vi "SMU simple tester.vi"() -> ()   [LabVIEW 2021]
uses:
  ctls/SMU status.ctl
  Source meter.lvlib
  <instrlib>/Keithley 2450/Keithley 2450.lvlib
  <userlib>/_MGI/1D Array/MGI Average/MGI Average (DBL[]).vi
  ctls/SMU settings.ctl
panel:
  out "Waveform Chart 2":dbl(graph)
  in  "Refresh Button":bool
  in  "VISA resource name 2":refnum<visa-resource-name>
  out "error":errorcluster
  out "Event Logger":string[](array[string])
  out "data":dbl[](array[numeric])
  out "SMU status":T1 {"Measure Function" items=["Volts", "Current", "Auto Resistance", "Manual Resistance", "Digitize Voltage", "Digitize Current"]; "Source Mode" items=["Voltage", "Current"]}
  out "Waveform Chart":dbl(graph)
  in  "Measurement settings":T2={"Source Mode "=1, "Source Level"=0.001, "Source Limit"=0.1, "Measure Function"=0, "Remote sense"=FALSE, "Clear buffer?"=FALSE, "Beep"=FALSE, "High Capacity"=FALSE, "Terminals"=0, "PLCs"=1.0, "Fast measurement"=FALSE} {"Measure Function" items=["Volts", "Current", "Auto Resistance", "Manual Resistance", "Digitize Voltage", "Digitize Current"]; "Source Mode" items=["Voltage", "Current"]; "Terminals" items=["Front", "Rear"]}
  in  "Disconnect":bool
  in  "Setup measuerment":bool
  in  "Start measurment":bool
  in  "Stop measurement":bool
  in  "End":bool
  in  "Connect":bool
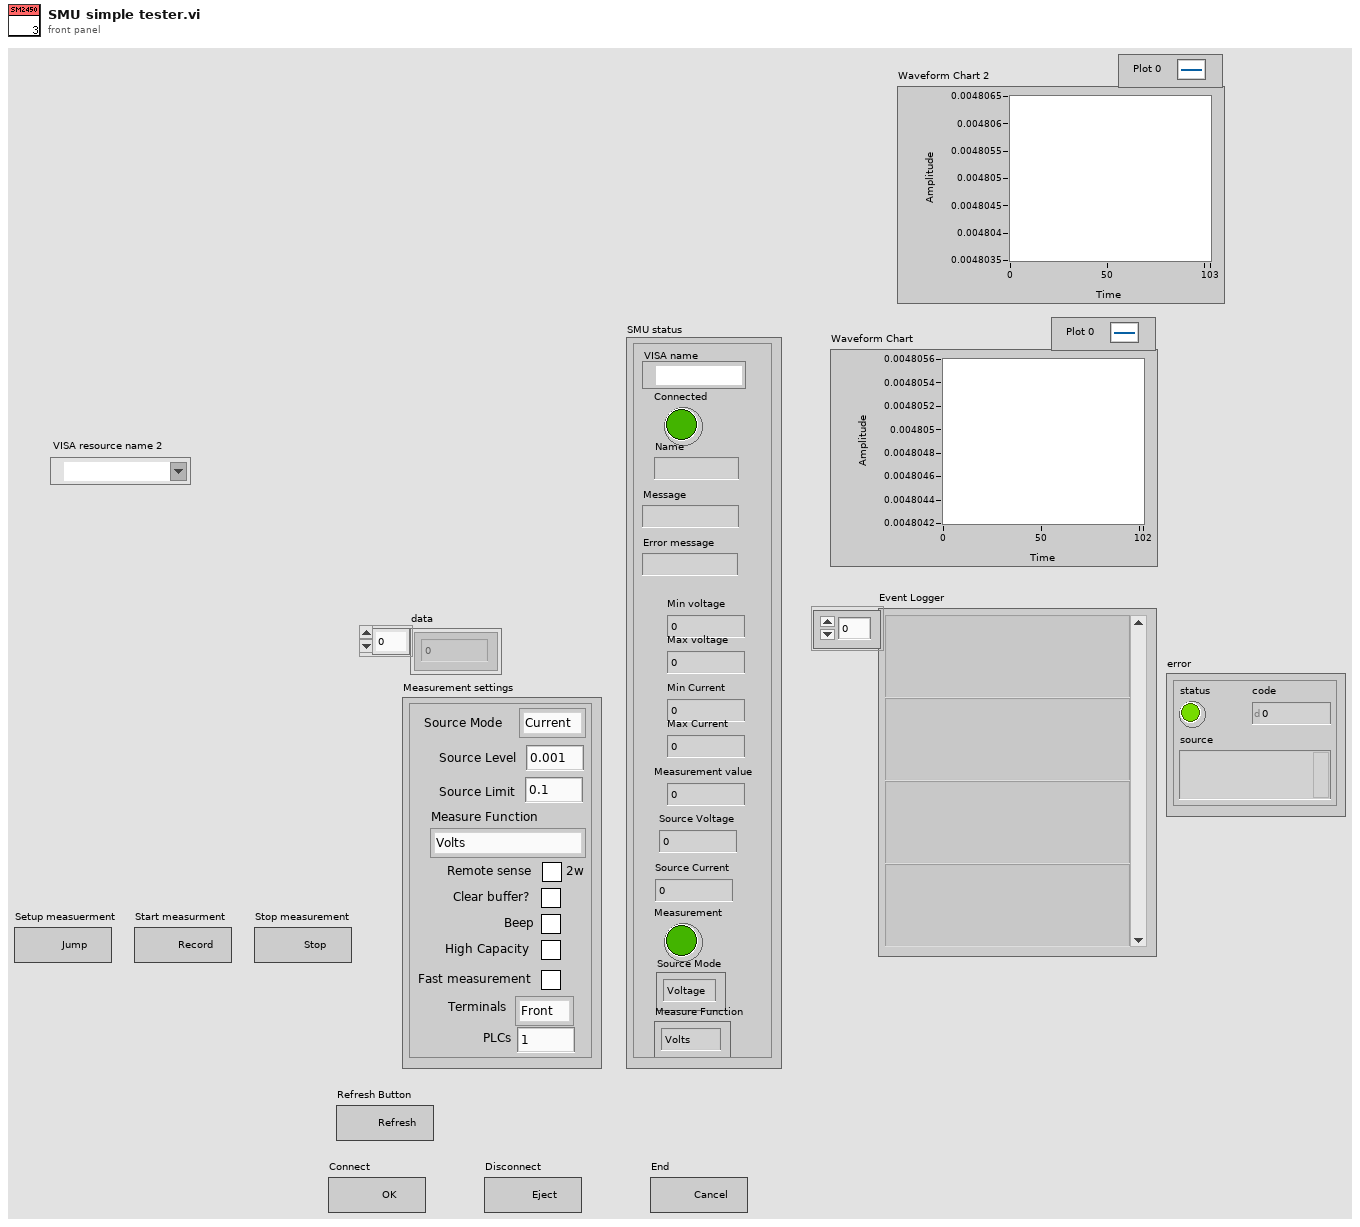
[diagram p1: front panel]
types:
  T1 = typedef "Source meter.lvlib/SMU status.ctl" = cluster{"VISA name":refnum<visa-resource-name>, "Connected":bool, "Name":string, "Message":string, "Error message":string, "Min voltage":dbl, "Max voltage":dbl, "Min Current":dbl, "Max Current":dbl, "Measurement value":dbl, "Source Voltage":dbl, "Measurement":bool, "Source Current":dbl, "Source Mode":u16, "Measure Function":u16}
  T2 = typedef "SMU settings.ctl" = cluster{"Source Mode ":u16, "Source Level":dbl, "Source Limit":dbl, "Measure Function":u16, "Remote sense":bool, "Clear buffer?":bool, "Beep":bool, "High Capacity":bool, "Terminals":u16, "PLCs":dbl, "Fast measurement":bool}
  T3 = cluster{"status":bool, "code":bool, "source":bool}
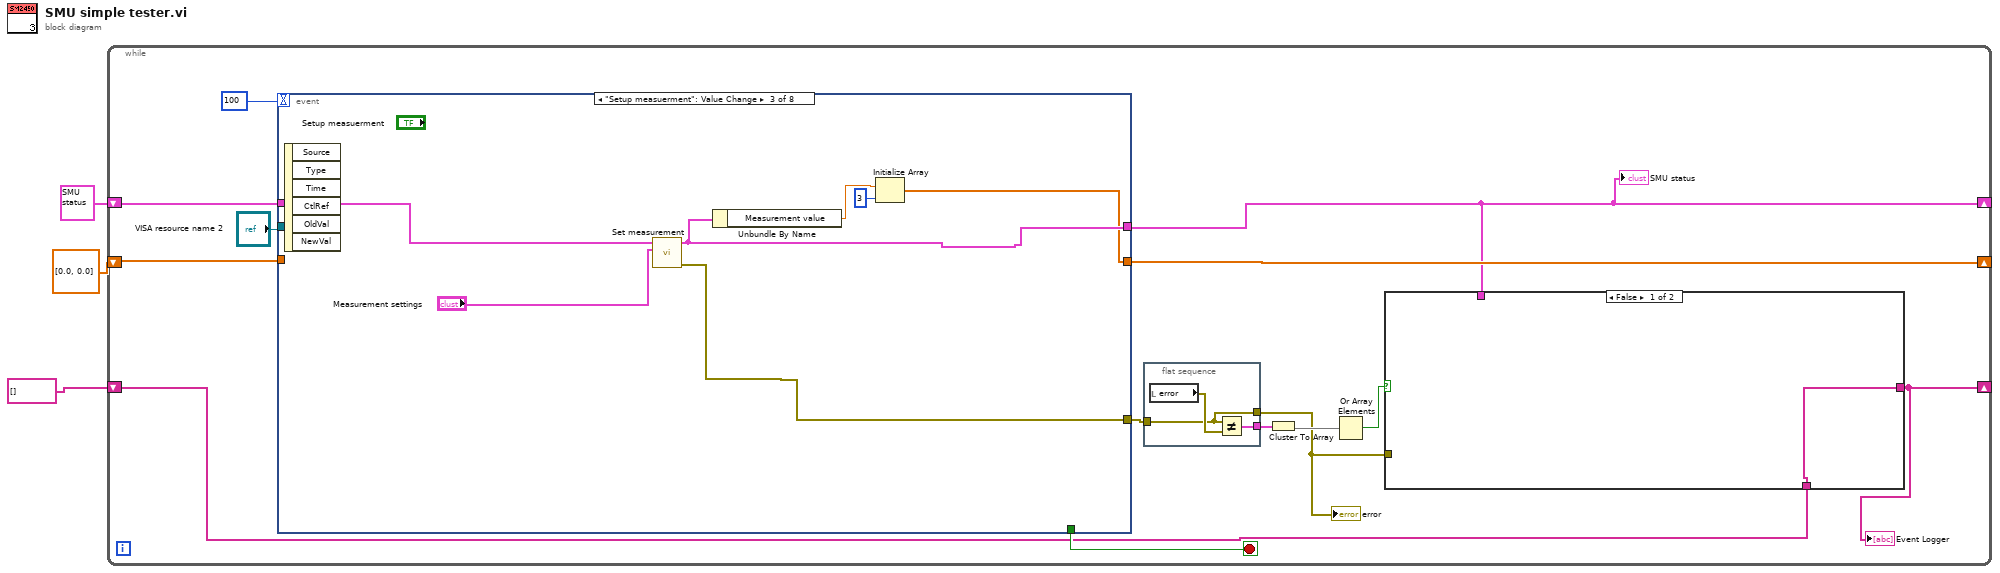
[diagram p0: block diagram]
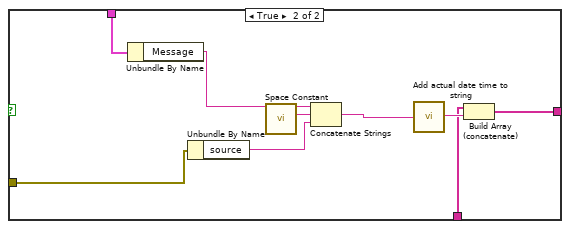
[diagram p2: hidden frame]
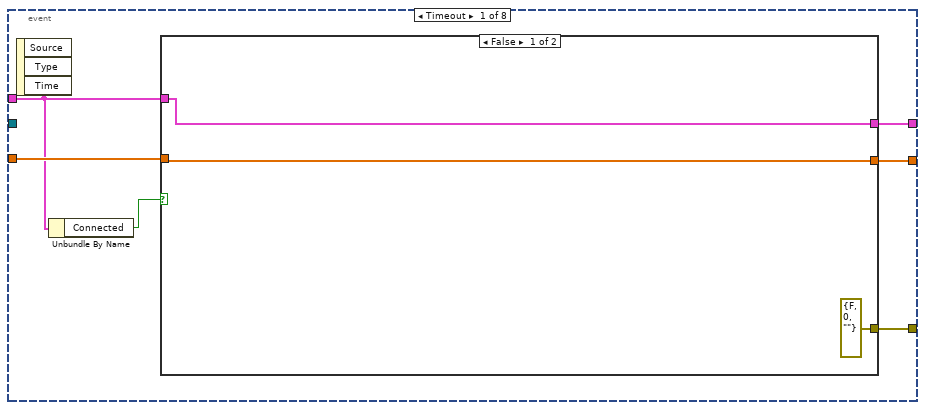
[diagram p3: hidden frame]
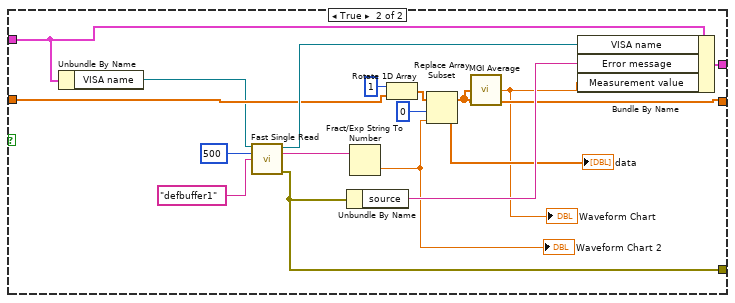
[diagram p4: hidden frame]
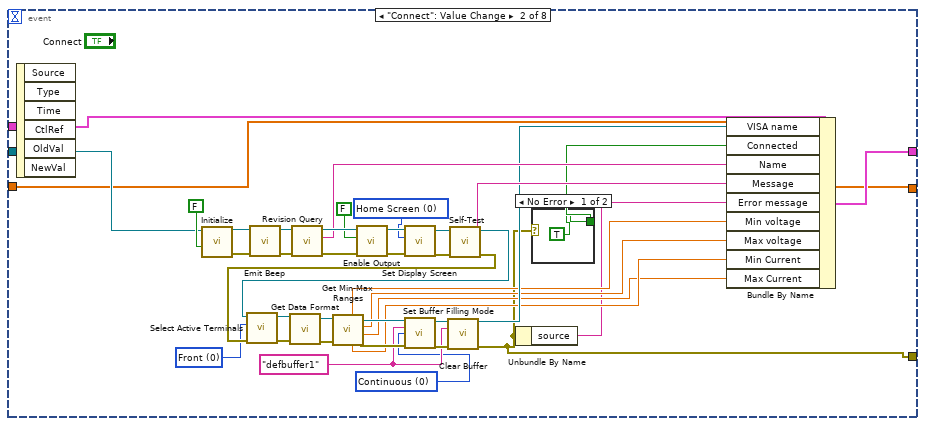
[diagram p5: hidden frame]
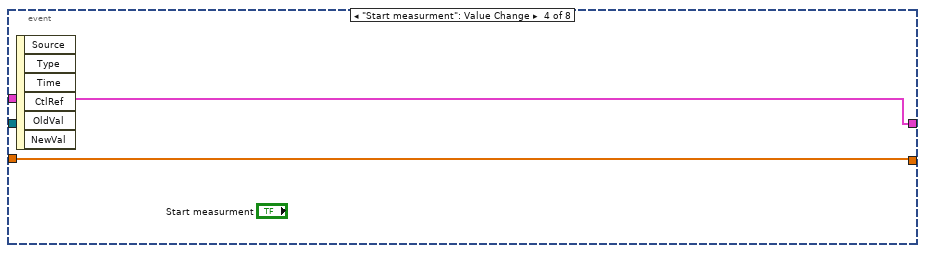
[diagram p7: hidden frame]
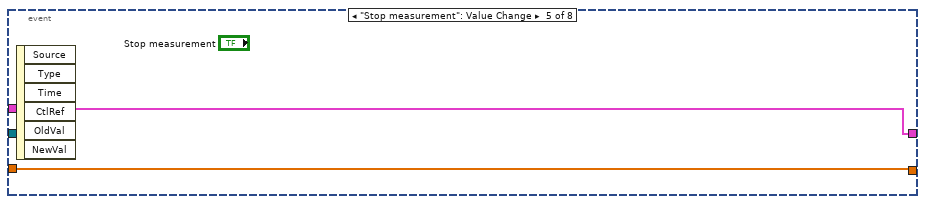
[diagram p8: hidden frame]
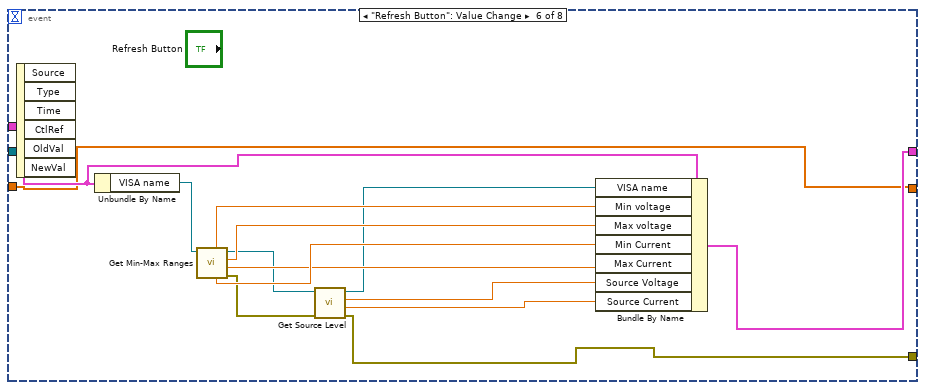
[diagram p9: hidden frame]
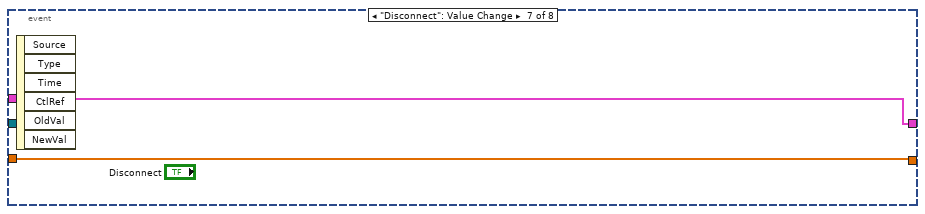
[diagram p10: hidden frame]
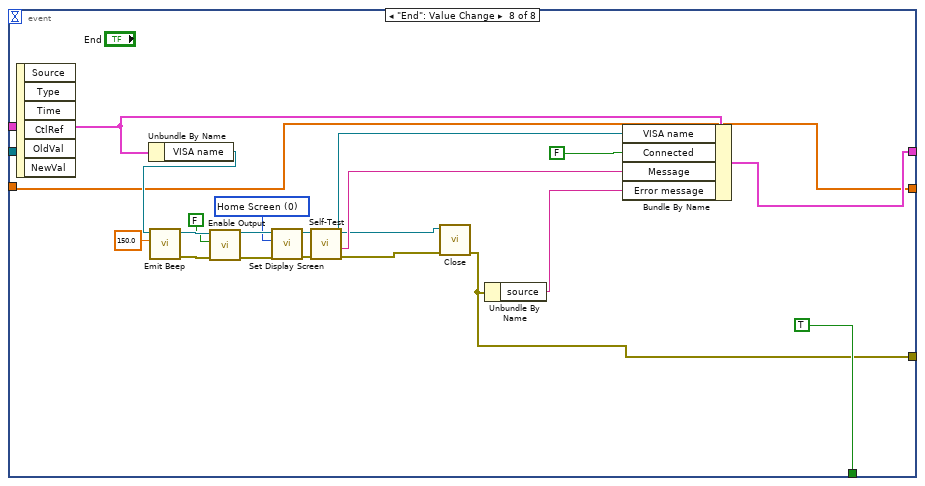
[diagram p11: hidden frame]
diagram:
  n1 = while {
    shift-right: [w4] -> _
    shift-left: T1 {"VISA name"="", "Connected"=FALSE, "Name"="", "Message"="", "Error message"="", "Min voltage"=0.0, "Max voltage"=0.0, "Min Current"=0.0, "Max Current"=0.0, "Measurement value"=0.0, "Source Voltage"=0.0, "Measurement"=FALSE, "Source Current"=0.0, "Source Mode"=0, "Measure Function"=0} ("SMU status") -> [w15]
    shift-right: [w13] -> _
    shift-left: dbl[] [0.0, 0.0] -> [w14]
    shift-right: [w6] -> _
    shift-left: string[] [] ("Event Logger") -> [w5]
    stop <- w16 stop-if-true
    n2 = event shown="[2] \"Setup measuerment\": Value Change" {
      selector: _ -> [_ _ _ _ _ _ _ _]
      dyn-events: _ -> [_ _ _ _ _ _ _ _]
      timeout: 100 -> [_ _ _ _ _ _ _ _]
      tunnel: [_ _ _ _ _ _ _ TRUE] -> w16
      tunnel: "VISA resource name 2" -> [_ w58 _ _ _ _ _ _]
      tunnel: w15 -> [w33 w59 w101 w105 w107 w111 w122 w127]
      tunnel: [w36 w60 w99 w105 w107 w110 w122 w126] -> w4
      tunnel: w14 -> [w35 w57 _ w104 w106 w109 w123 w125]
      tunnel: [w34 w57 w98 w104 w106 w109 w123 w125] -> w13
      tunnel: [w31 w56 w97 _ _ w108 _ w124] -> w11
      event Timeout {
        n3 = event-data() -> ()  [unwired: 1 in, 3 out]
        n4 = Unbundle By Name(w33) -> ("Connected"=w32:bool)
        n5 = case shown="False" w32 {
          tunnel: [w39 w47] -> w36
          tunnel: w35 -> [w38 w46]
          tunnel: [w38 w42] -> w34
          tunnel: w33 -> [w39 w45]
          tunnel: [errorcluster {"status"=FALSE, "code"=0, "source"=""} ("error out") w43] -> w31
          frame False {
          }
          frame True {
            n6 = Unbundle By Name(w45) -> ("VISA name"=w44:refnum<visa-resource-name>)
            n7 = call "Fast Single Read.vi"("VISA resource name"=w44, "Timeout (10000 ms)"=500, "Buffer Name (defbuffer1)"="defbuffer1") -> ("VISA resource name out"=w55:refnum<visa-resource-name>, "Data out"=w54:string, "error out"=w43:errorcluster)  [unwired: 10 in]
            n8 = Unbundle By Name(w43) -> ("source"=w53:string)
            n9 = Fract/Exp String To Number(string=w54) -> (number=w40:dbl)  [unwired: 3 in, 1 out]
            "Waveform Chart 2" <- w40
            n10 = Rotate 1D Array(1:w46, 2:1 ("n")) -> (0:w52:dbl[])
            n11 = Replace Array Subset(array=w52, new element=w40, index=0) -> (w42:dbl[])
            "data" <- w42
            n12 = call-poly <userlib>:"MGI Average.vi"("Double[]"=w42) -> ("Average"=w41:dbl)  [unwired: 1 in]
            "Waveform Chart" <- w41
            n13 = Bundle By Name(cluster=w45, "VISA name"=w55, "Error message"=w53, "Measurement value"=w41) -> (w47:T1)
          }
        }
      }
      event "Connect": Value Change {
        w66 = "defbuffer1" ("Buffer Name (defbuffer1)")
        w63 = u16 0 items=["Front", "Rear"] ("Active Terminals (0: Front)")
        w64 = u16 0 items=["Home Screen", "Source Screen", "Plot Screen", "User-defined Screen", "Statistics Screen", "Settings Screen", "Graph Screen", "Data sheet Screen"] ("Screen Home")
        w65 = u16 0 items=["Continuous", "Once"] ("Fill Type")
        n14 = event-data() -> ()  [unwired: 1 in, 6 out]
        n15 = call <instrlib>:"Initialize.vi"("Reset (True)"=FALSE, "VISA resource name"=w58) -> ("error out"=w94:errorcluster, "VISA resource name out"=w95:refnum<visa-resource-name>)  [unwired: 8 in]
        n16 = call <instrlib>:"Emit Beep.vi"("error in (no error)"=w94, "VISA resource name"=w95) -> ("error out"=w92:errorcluster, "VISA resource name out"=w93:refnum<visa-resource-name>)  [unwired: 8 in]
        n17 = call <instrlib>:"Revision Query.vi"("error in (no error)"=w92, "VISA resource name"=w93) -> ("error out"=w90:errorcluster, "Instrument Driver Revision"=w89:string, "VISA resource name out"=w91:refnum<visa-resource-name>)  [unwired: 6 in, 1 out]
        n18 = call <instrlib>:"Enable Output.vi"("error in (no error)"=w90, "Enable Output (T: Enable)"=FALSE, "VISA resource name"=w91) -> ("error out"=w87:errorcluster, "VISA resource name out"=w88:refnum<visa-resource-name>)  [unwired: 7 in]
        n19 = call <instrlib>:"Set Display Screen.vi"("error in (no error)"=w87, "Screen Home"=w64, "VISA resource name"=w88) -> ("error out"=w84:errorcluster, "VISA resource name out"=w85:refnum<visa-resource-name>)  [unwired: 7 in]
        n20 = call <instrlib>:"Self-Test.vi"("error in (no error)"=w84, "VISA resource name"=w85) -> ("error out"=w68:errorcluster, "Self-Test Result Message"=w86:string, "VISA resource name out"=w69:refnum<visa-resource-name>)  [unwired: 6 in, 1 out]
        n21 = call <instrlib>:"Select Active Terminals.vi"("error in (no error)"=w68, "Active Terminals (0: Front)"=w63, "VISA resource name"=w69) -> ("error out"=w82:errorcluster, "VISA resource name out"=w83:refnum<visa-resource-name>)  [unwired: 7 in]
        n22 = call <instrlib>:"Get Data Format.vi"("VISA resource name"=w83, "error in (no error)"=w82) -> ("VISA resource name out"=w81:refnum<visa-resource-name>, "error out"=w80:errorcluster)  [unwired: 11 in, 1 out]
        n23 = call <instrlib>:"Get Min-Max Ranges.vi"("error in (no error)"=w80, "VISA resource name"=w81) -> ("error out"=w78:errorcluster, "I Max"=w71:dbl, "V Max"=w73:dbl, "VISA resource name out"=w79:refnum<visa-resource-name>, "I Min"=w72:dbl, "V Min"=w74:dbl)  [unwired: 4 in]
        n24 = call <instrlib>:"Set Buffer Filling Mode.vi"("VISA resource name"=w79, "Buffer Name (defbuffer1)"=w66, "Fill Type"=w65, "error in (no error)"=w78) -> ("VISA resource name out"=w77:refnum<visa-resource-name>, "error out"=w76:errorcluster)  [unwired: 10 in]
        n25 = call <instrlib>:"Clear Buffer.vi"("VISA resource name"=w77, "Buffer Name (defbuffer1)"=w66, "error in (no error)"=w76) -> ("VISA resource name out"=w75:refnum<visa-resource-name>, "error out"=w56:errorcluster)  [unwired: 11 in]
        n26 = Unbundle By Name(w56) -> ("source"=w70:string)
        n27 = case shown="No Error" w56 {
          tunnel: [TRUE ("Connected") _] -> w67
          frame No Error {
          }
          frame Error {
          }
        }
        n28 = Bundle By Name(cluster=w59, "VISA name"=w75, "Connected"=w67, "Name"=w89, "Message"=w86, "Error message"=w70, "Min voltage"=w74, "Max voltage"=w73, "Min Current"=w72, "Max Current"=w71) -> (w60:T1)
      }
      event "Setup measuerment": Value Change {
        n29 = event-data() -> ()  [unwired: 1 in, 6 out]
        n30 = call "Set measurement.vi"("Measurement settings"="Measurement settings", "SMU status in"=w101) -> ("error out"=w97:errorcluster, "SMU status out"=w99:T1)  [unwired: 8 in]
        n31 = Unbundle By Name(w99) -> ("Measurement value"=w103:dbl)
        n32 = Initialize Array(w103, 3 ("dimension size")) -> (w98:dbl[])
      }
      event "Start measurment": Value Change {
        n33 = event-data() -> ()  [unwired: 1 in, 6 out]
      }
      event "Stop measurement": Value Change {
        n34 = event-data() -> ()  [unwired: 1 in, 6 out]
      }
      event "Refresh Button": Value Change {
        n35 = event-data() -> ()  [unwired: 1 in, 6 out]
        n36 = Unbundle By Name(w111) -> ("VISA name"=w121:refnum<visa-resource-name>)
        n37 = call <instrlib>:"Get Min-Max Ranges.vi"("VISA resource name"=w121) -> ("error out"=w114:errorcluster, "I Max"=w117:dbl, "V Max"=w119:dbl, "VISA resource name out"=w116:refnum<visa-resource-name>, "I Min"=w118:dbl, "V Min"=w120:dbl)  [unwired: 5 in]
        n38 = call <instrlib>:"Get Source Level.vi"("error in (no error)"=w114, "VISA resource name"=w116) -> ("error out"=w108:errorcluster, "Current Level Out"=w113:dbl, "Voltage Level Out"=w112:dbl, "VISA resource name out"=w115:refnum<visa-resource-name>)  [unwired: 6 in]
        n39 = Bundle By Name(cluster=w111, "VISA name"=w115, "Min voltage"=w120, "Max voltage"=w119, "Min Current"=w118, "Max Current"=w117, "Source Voltage"=w112, "Source Current"=w113) -> (w110:T1)
      }
      event "Disconnect": Value Change {
        n40 = event-data() -> ()  [unwired: 1 in, 6 out]
      }
      event "End": Value Change {
        w130 = u16 0 items=["Home Screen", "Source Screen", "Plot Screen", "User-defined Screen", "Statistics Screen", "Settings Screen", "Graph Screen", "Data sheet Screen"] ("Screen Home")
        n41 = event-data() -> ()  [unwired: 1 in, 6 out]
        n42 = Unbundle By Name(w127) -> ("VISA name"=w133:refnum<visa-resource-name>)
        n43 = call <instrlib>:"Emit Beep.vi"("Beep Frequency (300)"=150.0, "VISA resource name"=w133) -> ("error out"=w141:errorcluster, "VISA resource name out"=w142:refnum<visa-resource-name>)  [unwired: 8 in]
        n44 = call <instrlib>:"Enable Output.vi"("error in (no error)"=w141, "Enable Output (T: Enable)"=FALSE, "VISA resource name"=w142) -> ("error out"=w139:errorcluster, "VISA resource name out"=w140:refnum<visa-resource-name>)  [unwired: 7 in]
        n45 = call <instrlib>:"Set Display Screen.vi"("error in (no error)"=w139, "Screen Home"=w130, "VISA resource name"=w140) -> ("error out"=w136:errorcluster, "VISA resource name out"=w137:refnum<visa-resource-name>)  [unwired: 7 in]
        n46 = call <instrlib>:"Self-Test.vi"("error in (no error)"=w136, "VISA resource name"=w137) -> ("error out"=w134:errorcluster, "Self-Test Result Message"=w138:string, "VISA resource name out"=w135:refnum<visa-resource-name>)  [unwired: 6 in, 1 out]
        n47 = call <instrlib>:"Close.vi"("error in (no error)"=w134, "VISA resource name"=w135) -> ("error out"=w124:errorcluster)  [unwired: 9 in]
        n48 = Unbundle By Name(w124) -> ("source"=w132:string)
        n49 = Bundle By Name(cluster=w127, "VISA name"=w135, "Connected"=FALSE, "Message"=w138, "Error message"=w132) -> (w126:T1)
      }
    }
    "SMU status" <- w4
    n50 = flat-sequence {
      tunnel: w11 -> [w29]
      tunnel: [w29] -> w7
      tunnel: [w28] -> w10
      frame #0 {
        n51 = local read "error"() -> (w30:errorcluster)
        n52 = Not Equal?(x=w29, y=w30) -> (x != y?=w28:T3)
      }
    }
    n53 = Cluster To Array(cluster=w10) -> (array=w9:bool[])
    n54 = Or Array Elements(Boolean array=w9) -> (logical OR=w8:bool)
    n55 = case shown="False" w8 {
      tunnel: [w18 w27] -> w6
      tunnel: w7 -> [_ w22]
      tunnel: w4 -> [_ w21]
      tunnel: w5 -> [w18 w19]
      frame False {
      }
      frame True {
        n56 = Unbundle By Name(w21) -> ("Message"=w20:string)
        n57 = Unbundle By Name(w22) -> ("source"=w23:string)
        n58 = call <vilib>:"Space Constant.vi"() -> ("String"=w24:string)
        n59 = Concatenate Strings(w20, w24, w23) -> (w25:string)
        n60 = call "Add actual date time to string.vi"("String in"=w25) -> ("String out"=w26:string)  [unwired: 4 in]
        n61 = Build Array (concatenate)(w19, w26) -> (w27:string[])
      }
    }
    "Event Logger" <- w6
    "error" <- w7
  }
